vi "json To Pretty String - array path.vi"(8 "error in (no error)":errorcluster, 10 "path":string[](array[string]), 11 "JSON Document in":refnum<class "JSON Document.lvclass">) -> (0 "error out":errorcluster, 2 "json string":string, 3 "JSON Document out":refnum<class "JSON Document.lvclass">)   [LabVIEW 2015, in "JSON Document.lvclass"]
uses:
  JSON Document.lvclass
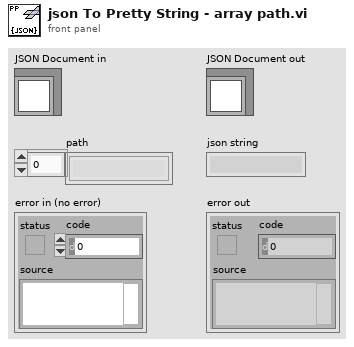
[diagram p1: front panel]
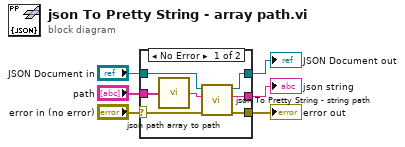
[diagram p0: block diagram]
diagram:
  n1 = case shown="No Error" "error in (no error)" {
    selector: "error in (no error)" -> [w9 w15]
    tunnel: [w8 w15] -> w5
    tunnel: [w12 w14] -> w3
    tunnel: "JSON Document in" -> [w13 w14]
    tunnel: [w7 _] -> w2
    tunnel: "path" -> [w10 _]
    frame No Error {
      n2 = call "json path array to path.vi"("path"=w10) -> ("String"=w11:string)
      n3 = call "json To Pretty String - string path.vi"("error in (no error)"=w9, "path"=w11, "JSON Document in"=w13) -> ("error out"=w8:errorcluster, "json string"=w7:string, "JSON Document out"=w12:refnum<class "JSON Document.lvclass">)  [unwired: 6 in]
    }
    frame Error {
    }
  }
  "error out" <- w5
  "JSON Document out" <- w3
  "json string" <- w2
